vi "Initialize Front Panel.vi"(8 "error in (no error)":errorcluster, 11 "Popup View in":refnum<class "Popup View.lvclass">) -> (0 "error out":errorcluster, 3 "Popup View out":refnum<class "Popup View.lvclass">)   [LabVIEW 2017, in "Popup View.lvclass"]
doc: "<License>\nCopyright © 2017 Composed Systems, LLC | All rights reserved\nwww.composed.io\n\nAuthor: Ethan Stern <ethan.stern@composed.io>\n\nThis software is provided \"AS IS\" WITHOUT WARRANTIES, either express or implied, AND IS FOR EDUCATIONAL PURPOSES ONLY.\n</License>"
uses:
  <vilib>/gpm_packages/@cs/popup-viewmanager/Example/Popup View/Popup View.lvclass
  C:/Program Files/National Instruments/LabVIEW 2017/vi.lib/gpm_packages/@cs/popup-viewmanager/Source/Popup ViewManager/Popup ViewManager.lvclass
  <vilib>/gpm_packages/@cs/popup-viewmanager/Example/Popup View/Popup View.lvclass/Popup View.ctl
  <vilib>/gpm_packages/@cs/mva-viewable/Source/IViewable/IViewable Messages/Insert Front Panel Msg/Insert Front Panel Msg.lvclass/Insert Front Panel Msg.ctl
  <vilib>/ActorFramework/Message Enqueuer/Message Enqueuer.lvclass/Message Enqueuer.ctl
  <vilib>/ActorFramework/Message Enqueuer/Enqueue.vi
  <vilib>/gpm_packages/@cs/mva-viewable/Source/IViewable/IViewable Messages/Insert Front Panel Msg/Insert Front Panel Msg.lvclass
  C:/Program Files/National Instruments/LabVIEW 2017/vi.lib/ActorFramework/Message/Message.lvclass
  <vilib>/ActorFramework/Message Priority Queue/Priority Enqueue.vi
  <vilib>/gpm_packages/@cs/popup-viewmanager/Source/Popup ViewManager/Popup ViewManager.lvclass
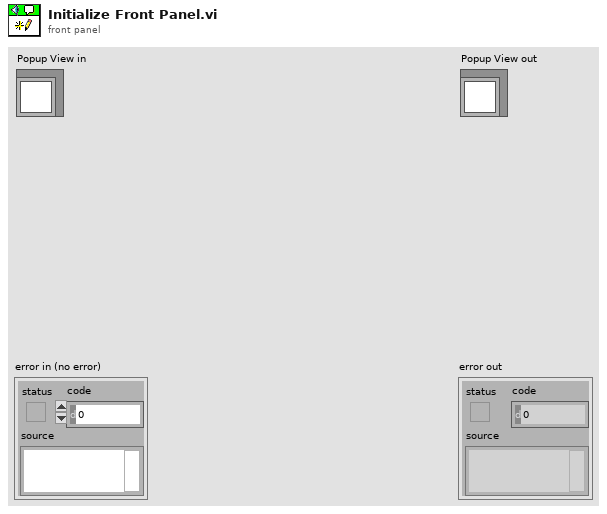
[diagram p1: front panel]
types:
  T1 = typedef "IViewable.lvlib/ProtectedSubpanel.lvclass/Protected Subpanel Reference.ctl" = refnum<data-value>
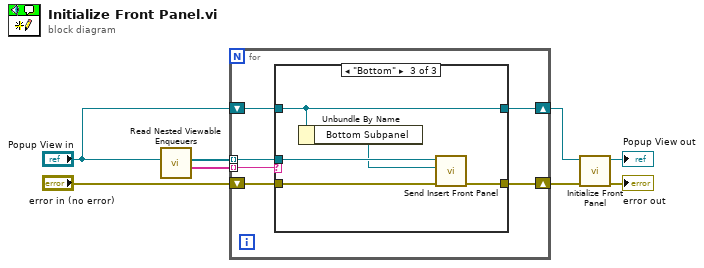
[diagram p0: block diagram]
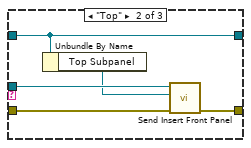
[diagram p3: hidden frame]
diagram:
  n1 = call <vilib>:"Read Nested Viewable Enqueuers.vi"("Popup ViewManager in"="Popup View in") -> ("Viewable Names"=w3:string[], "Nested Enqueuers"=w4:refnum<class "Message Enqueuer.lvclass">[])  [unwired: 9 in]
  n2 = for {
    shift-right: [w13] -> w5
    shift-left: "error in (no error)" -> [w14]
    tunnel: w4 -> [w11] mode=indexing
    tunnel: w3 -> [w12] mode=indexing
    shift-right: [w9] -> w1
    shift-left: "Popup View in" -> [w10]
    n3 = case shown="\"Bottom\"" w12 {
      tunnel: [w15 w19 w24] -> w13
      tunnel: w14 -> [w15 w20 w25]
      tunnel: w11 -> [_ w18 w23]
      tunnel: w10 -> [w16 w21 w26]
      tunnel: [w16 w21 w26] -> w9
      frame Default {
      }
      frame "Top" {
        n4 = Unbundle By Name(w21) -> ("Top Subpanel"=w17:T1)
        n5 = call <vilib>:"Send Insert Front Panel.vi"("error in (no error)"=w20, "Protected Subpanel"=w17, "Message Enqueuer"=w18) -> ("error out"=w19:errorcluster)  [unwired: 7 in, 1 out]
      }
      frame "Bottom" {
        n6 = Unbundle By Name(w26) -> ("Bottom Subpanel"=w22:T1)
        n7 = call <vilib>:"Send Insert Front Panel.vi"("error in (no error)"=w25, "Protected Subpanel"=w22, "Message Enqueuer"=w23) -> ("error out"=w24:errorcluster)  [unwired: 7 in, 1 out]
      }
    }
  }
  n8 = call-parent "Initialize Front Panel.vi"("error in (no error)"=w5, "IViewable in"=w1) -> ("error out"=→"error out":errorcluster, "IViewable out"=→"Popup View out":refnum<class "Popup View.lvclass">)  [unwired: 8 in]
